vi "TC_R_VtoC.vi"(11 "Thermocouple Voltage":dbl caption="热电偶电压" format="%0.6f") -> (3 "T(c)":dbl format="%#_16f")   [LabVIEW 2012]
doc: "功能：\n\nR型热电偶电压转换为摄氏度。\n\ncsxcs_366创建。"
uses:
  <vilib>/Analysis/polynomials.llb/Scalar Polynomial Evaluation (DBL).vi
  <vilib>/Analysis/NI_AALPro.lvlib
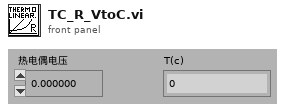
[diagram p1: front panel]
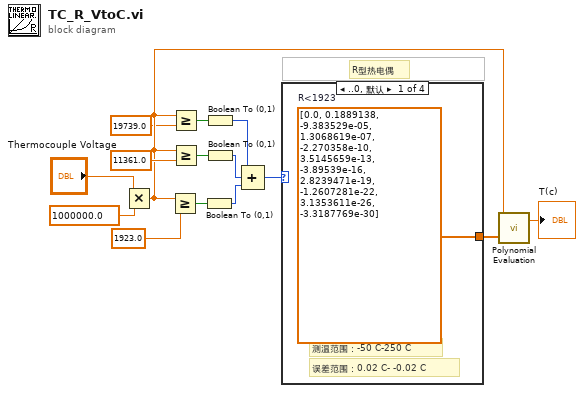
[diagram p0: block diagram]
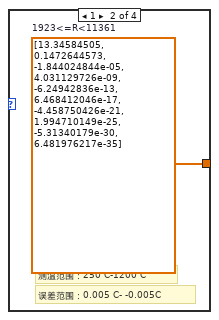
[diagram p2: hidden frame]
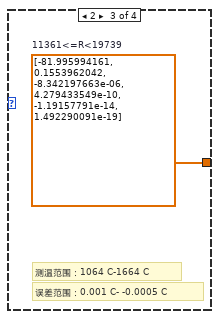
[diagram p3: hidden frame]
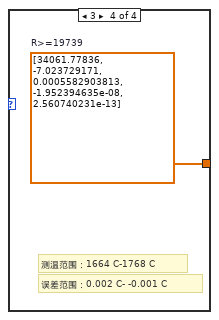
[diagram p4: hidden frame]
diagram:
  # "R型热电偶"
  n1 = Multiply(x="Thermocouple Voltage", y=1000000.0) -> (x*y=w2:dbl)
  n2 = Greater Or Equal?(x=w2, y=1923.0) -> (x >= y?=w9:bool)
  n3 = Greater Or Equal?(x=w2, y=19739.0) -> (x >= y?=w5:bool)
  n4 = Greater Or Equal?(x=w2, y=11361.0) -> (x >= y?=w10:bool)
  n5 = Boolean To (0,1)(Boolean=w9) -> (0, 1=w8:i16)
  n6 = Boolean To (0,1)(Boolean=w5) -> (0, 1=w4:i16)
  n7 = Boolean To (0,1)(Boolean=w10) -> (0, 1=w7:i16)
  n8 = Compound Arithmetic op=ADD(w4, w7, w8) -> (w6:i16)
  n9 = case shown="..0, 默认" w6 {
    tunnel: [w16 w17 w18 w19] -> w3
    frame ..0, Default {
      w16 = dbl[] [0.0, 0.1889138, -9.383529e-05, 1.3068619e-07, -2.270358e-10, 3.5145659e-13, -3.89539e-16, 2.8239471e-19, -1.2607281e-22, 3.1353611e-26, -3.3187769e-30]  # R<1923
      # "误差范围：0.02 C- -0.02 C"
      # "测温范围：-50 C-250 C"
    }
    frame 1 {
      w17 = dbl[] [13.34584505, 0.1472644573, -1.844024844e-05, 4.031129726e-09, -6.24942836e-13, 6.468412046e-17, -4.458750426e-21, 1.994710149e-25, -5.31340179e-30, 6.481976217e-35]  # 1923<=R<11361
      # "误差范围：0.005 C- -0.005C"
      # "测温范围：250 C-1200 C"
    }
    frame 2 {
      w18 = dbl[] [-81.995994161, 0.1553962042, -8.342197663e-06, 4.279433549e-10, -1.19157791e-14, 1.492290091e-19]  # 11361<=R<19739
      # "误差范围：0.001 C- -0.0005 C"
      # "测温范围：1064 C-1664 C"
    }
    frame 3 {
      w19 = dbl[] [34061.77836, -7.023729171, 0.0005582903813, -1.952394635e-08, 2.560740231e-13]  # R>=19739
      # "误差范围：0.002 C- -0.001 C"
      # "测温范围：1664 C-1768 C"
    }
  }
  n10 = call-poly <vilib>:"Polynomial Evaluation.vi"("P(x)"=w3, "a"=w2) -> ("P(a)"=→"T(c)":dbl)  [unwired: 1 out]
